vi "5492_WPI_JoystickArcadeMapping.vi"(6 "Max Output":dbl=1.0, 7 "Square Inputs":bool=TRUE, 8 "Slow Toggle":bool, 9 "Y axis value":dbl, 10 "X axis value":dbl, 11 "Orientation Toggle":bool) -> (1 "Right Motor Value":dbl, 2 "Left Motor Value":dbl)   [LabVIEW 2017]
doc: "Uses a standard algorithm to map joystick axes into motor updates for arcade driving. This algorithm does not saturate over half of the range.\n\nThis software is licensed. Open the labview\\readme\\WPI Robotics Library Open Source License.txt file for more information."
uses:
  5492_OrientationButtonPress.vi
  5492_DriveOrientation.vi
  5492_SlowButton.vi
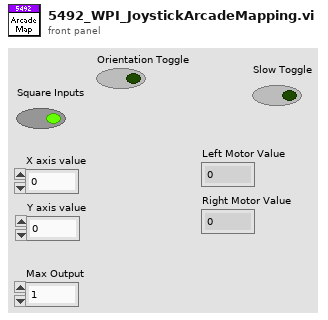
[diagram p1: front panel]
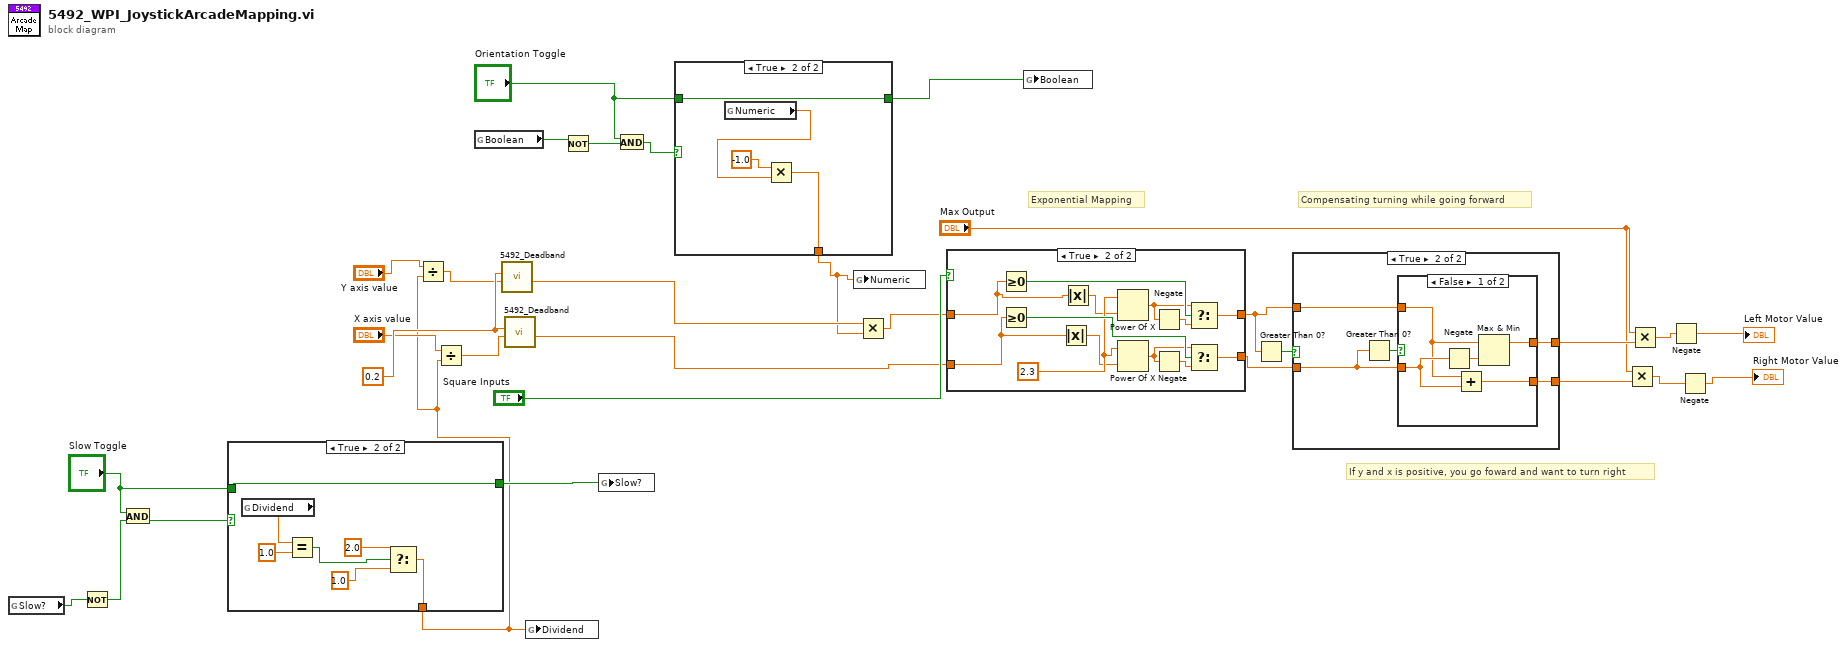
[diagram p0: block diagram]
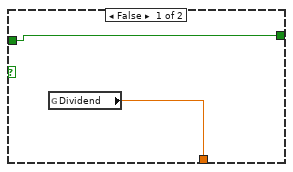
[diagram p2: hidden frame]
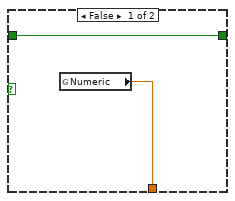
[diagram p3: hidden frame]
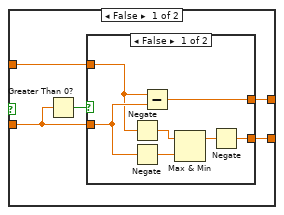
[diagram p4: hidden frame]
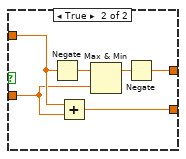
[diagram p5: hidden frame]
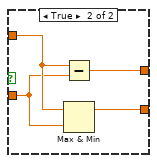
[diagram p6: hidden frame]
diagram:
  w24 = 0.2
  # "Compensating turning while going forward"
  # "Exponential Mapping"
  # "If y and x is positive, you go foward and want to turn right"
  n1 = global read "5492_SlowButton.vi" "Slow?"() -> (w6:bool)
  n2 = Not(x=w6) -> (.not. x?=w7:bool)
  n3 = And(x="Slow Toggle", y=w7) -> (x .and. y?=w10:bool)
  n4 = case shown="True" w10 {
    tunnel: "Slow Toggle" -> [w33 w40]
    tunnel: [w33 w40] -> w8
    tunnel: [w32 w37] -> w1
    frame False {
      n5 = global read "5492_SlowButton.vi" "Dividend"() -> (w32:dbl)
    }
    frame True {
      n6 = global read "5492_SlowButton.vi" "Dividend"() -> (w35:dbl)
      n7 = Equal?(x=w35, y=1.0) -> (x = y?=w36:bool)
      n8 = Select(t=2.0, s=w36, f=1.0) -> (s? t:f=w37:dbl)
    }
  }
  n9 = Divide(x="Y axis value", y=w1) -> (x/y=w4:dbl)
  n10 = Divide(x="X axis value", y=w1) -> (x/y=w3:dbl)
  n11 = global read "5492_OrientationButtonPress.vi" "Boolean"() -> (w17:bool)
  n12 = call "5492_Deadband.vi"("Input"=w4, "DeadBand"=w24) -> ("Output"=w19:dbl)  [unwired: 9 in]
  n13 = call "5492_Deadband.vi"("Input"=w3, "DeadBand"=w24) -> ("Output"=w11:dbl)  [unwired: 9 in]
  n14 = global write "5492_SlowButton.vi" "Dividend"(w1) -> ()
  n15 = Not(x=w17) -> (.not. x?=w14:bool)
  n16 = global write "5492_SlowButton.vi" "Slow?"(w8) -> ()
  n17 = And(x="Orientation Toggle", y=w14) -> (x .and. y?=w16:bool)
  n18 = case shown="True" w16 {
    tunnel: [w42 w44] -> w12
    tunnel: "Orientation Toggle" -> [w41 w43]
    tunnel: [w41 w43] -> w15
    frame False {
      n19 = global read "5492_DriveOrientation.vi" "Numeric"() -> (w42:dbl)
    }
    frame True {
      n20 = global read "5492_DriveOrientation.vi" "Numeric"() -> (w45:dbl)
      n21 = Multiply(x=-1.0, y=w45) -> (x*y=w44:dbl)
    }
  }
  n22 = global write "5492_DriveOrientation.vi" "Numeric"(w12) -> ()
  n23 = Multiply(x=w19, y=w12) -> (x*y=w18:dbl)
  n24 = case shown="True" "Square Inputs" {
    tunnel: [w47 w61] -> w29
    tunnel: [w48 w60] -> w30
    tunnel: w11 -> [w47 w51]
    tunnel: w18 -> [w48 w49]
    frame False {
    }
    frame True {
      w53 = 2.3
      n25 = Greater Or Equal To 0?(x=w49) -> (x >= 0?=w56:bool)
      n26 = Greater Or Equal To 0?(x=w51) -> (x >= 0?=w59:bool)
      n27 = Absolute Value(x=w51) -> (abs(x)=w52:dbl)
      n28 = Absolute Value(x=w49) -> (abs(x)=w50:dbl)
      n29 = Power Of X(1:w50, 2:w53) -> (0:w54:dbl)
      n30 = Power Of X(1:w52, 2:w53) -> (0:w55:dbl)
      n31 = Negate(x=w54) -> (-x=w57:dbl)
      n32 = Negate(x=w55) -> (-x=w58:dbl)
      n33 = Select(t=w54, s=w56, f=w57) -> (s? t:f=w60:dbl)
      n34 = Select(t=w55, s=w59, f=w58) -> (s? t:f=w61:dbl)
    }
  }
  n35 = global write "5492_OrientationButtonPress.vi" "Boolean"(w15) -> ()
  n36 = Greater Than 0?(x=w30) -> (x > 0?=w31:bool)
  n37 = case shown="True" w31 {
    tunnel: w29 -> [w65 w83]
    tunnel: w30 -> [w64 w82]
    tunnel: [w63 w81] -> w28
    tunnel: [w62 w80] -> w27
    frame False {
      n38 = Greater Than 0?(x=w65) -> (x > 0?=w66:bool)
      n39 = case shown="False" w66 {
        tunnel: w65 -> [w73 w75]
        tunnel: w64 -> [w71 w76]
        tunnel: [w67 w77] -> w63
        tunnel: [w68 w74] -> w62
        frame False {
          n40 = Negate(x=w71) -> (-x=w72:dbl)
          n41 = Negate(x=w73) -> (-x=w70:dbl)
          n42 = Subtract(x=w71, y=w73) -> (x-y=w67:dbl)
          n43 = Max & Min(x=w72, y=w70) -> (max(x,y)=w69:dbl)  [unwired: 1 out]
          n44 = Negate(x=w69) -> (-x=w68:dbl)
        }
        frame True {
          n45 = Negate(x=w76) -> (-x=w79:dbl)
          n46 = Add(x=w76, y=w75) -> (x+y=w74:dbl)
          n47 = Max & Min(x=w79, y=w75) -> (max(x,y)=w78:dbl)  [unwired: 1 out]
          n48 = Negate(x=w78) -> (-x=w77:dbl)
        }
      }
    }
    frame True {
      n49 = Greater Than 0?(x=w83) -> (x > 0?=w84:bool)
      n50 = case shown="False" w84 {
        tunnel: w83 -> [w89 w91]
        tunnel: w82 -> [w86 w92]
        tunnel: [w87 w90] -> w81
        tunnel: [w85 w93] -> w80
        frame False {
          n51 = Negate(x=w89) -> (-x=w88:dbl)
          n52 = Add(x=w86, y=w89) -> (x+y=w85:dbl)
          n53 = Max & Min(x=w86, y=w88) -> (max(x,y)=w87:dbl)  [unwired: 1 out]
        }
        frame True {
          n54 = Subtract(x=w92, y=w91) -> (x-y=w90:dbl)
          n55 = Max & Min(x=w92, y=w91) -> (max(x,y)=w93:dbl)  [unwired: 1 out]
        }
      }
    }
  }
  n56 = Multiply(x="Max Output", y=w27) -> (x*y=w23:dbl)
  n57 = Multiply(x="Max Output", y=w28) -> (x*y=w20:dbl)
  n58 = Negate(x=w20) -> (-x=→"Left Motor Value":dbl)
  n59 = Negate(x=w23) -> (-x=→"Right Motor Value":dbl)
